vi "Global 1.vi"() -> ()   [LabVIEW 2017]
panel:
  out "PLC Comm stat":bool
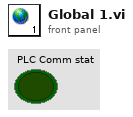
[diagram p1: front panel]
diagram:
